vi "Send SLM_DeInit_Done.vi"(7 "Message Priority (Normal)":T1=enum."Normal", 8 "error in (no error)":errorcluster, 10 "Variant":variant, 11 "Message Enqueuer":refnum<class "Message Enqueuer.lvclass">) -> (0 "error out":errorcluster, 3 "Message Enqueuer out":refnum<class "Message Enqueuer.lvclass">)   [LabVIEW 2023, in "SLMLibrary.lvlib" / "SLMComm.lvlib" / "SLM_DeInit_Done Msg.lvclass"]
doc: "This VI sends the message to an actor."
uses:
  SLM_DeInit_Done Msg.lvclass
  <vilib>/ActorFramework/Message Enqueuer/Message Enqueuer.lvclass
  <vilib>/ActorFramework/Message Enqueuer/Message Priority.ctl
  SLM_DeInit_Done Msg.lvclass/SLM_DeInit_Done Msg.ctl
  <vilib>/ActorFramework/Message Enqueuer/Message Enqueuer.lvclass/Message Enqueuer.ctl
  <vilib>/ActorFramework/Message Priority Queue/Priority Enqueue.vi
  C:/Program Files/National Instruments/LabVIEW 2023/vi.lib/ActorFramework/Message/Message.lvclass
  C:/Users/quantum/Documents/LVDAQ/Interfaces/AbstractInstrumentClasses/SLM_LV/SLMComm Messages/SLM_DeInit_Done Msg/SLM_DeInit_Done Msg.lvclass
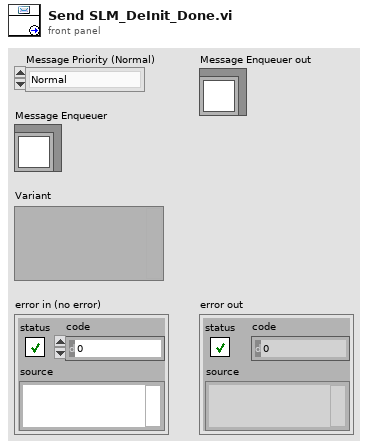
[diagram p1: front panel]
types:
  T1 = typedef "Actor Framework.lvlib/Message Enqueuer.lvclass/Message Priority.ctl" = enum16{"Low", "Normal", "High"}
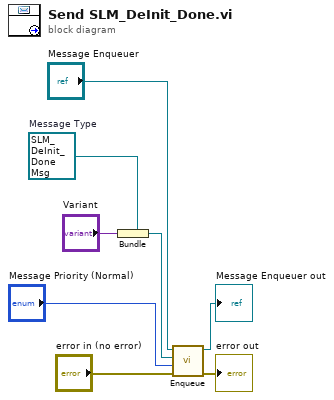
[diagram p0: block diagram]
diagram:
  w5 = refnum<class "SLM_DeInit_Done Msg.lvclass"> refnum  # Message Type
  n1 = Bundle(cluster=w5, "Variant") -> (w4:refnum<class "SLM_DeInit_Done Msg.lvclass">)
  n2 = call <vilib>:"Enqueue.vi"("error in (no error)"="error in (no error)", "Message Priority (Normal)"="Message Priority (Normal)", "Message"=w4, "Message Enqueuer in"="Message Enqueuer") -> ("error out"=→"error out":errorcluster, "Message Enqueuer in"=→"Message Enqueuer out":refnum<class "Message Enqueuer.lvclass">)  [unwired: 6 in]
